vi "TP1.4.vi"() -> ()   [LabVIEW 2013]
panel:
  out "Waveform Graph 2":dbl[](graph)
  in  "Frecuencia":dbl=5.0
  in  "Amplitud":dbl=10.0
  in  "Cantidad de Muestras":i32=1000
  in  "Boolean":bool
  in  "Función":T1(ring)
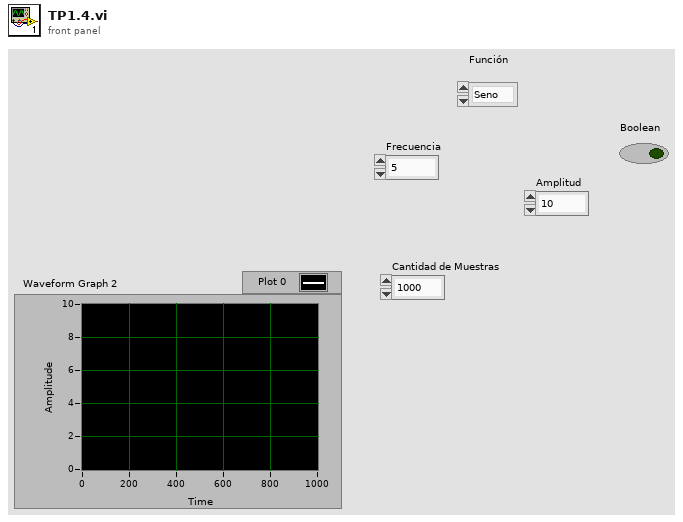
[diagram p1: front panel]
types:
  T1 = enum16{"Seno", "Rampa", "Triangular", "Cuadrada"}
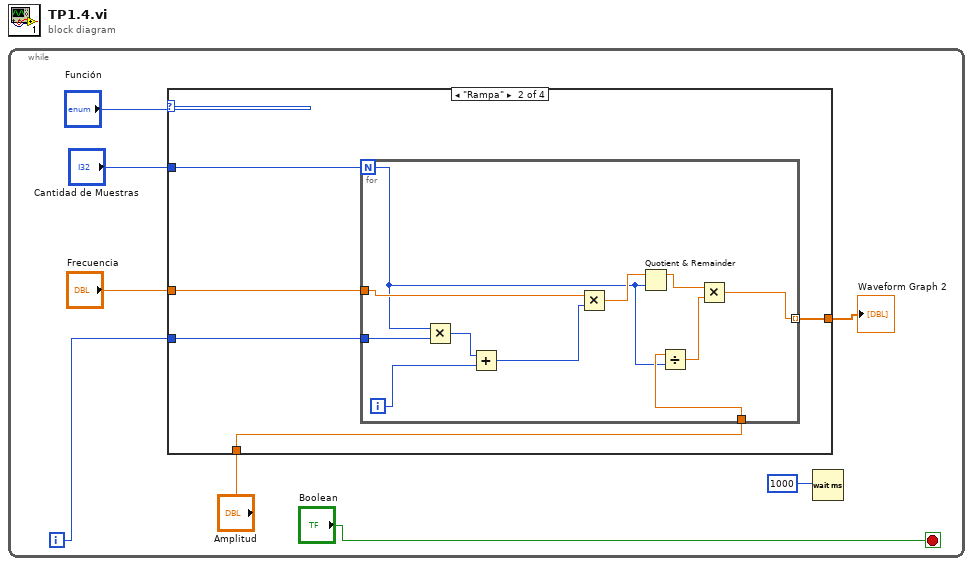
[diagram p0: block diagram]
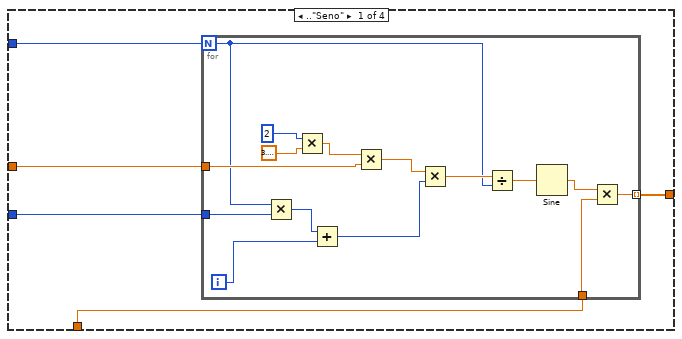
[diagram p2: hidden frame]
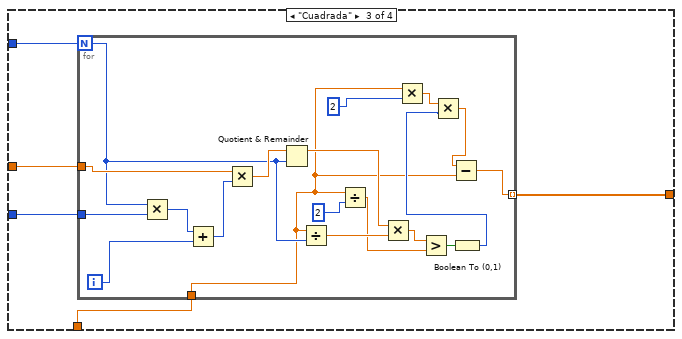
[diagram p3: hidden frame]
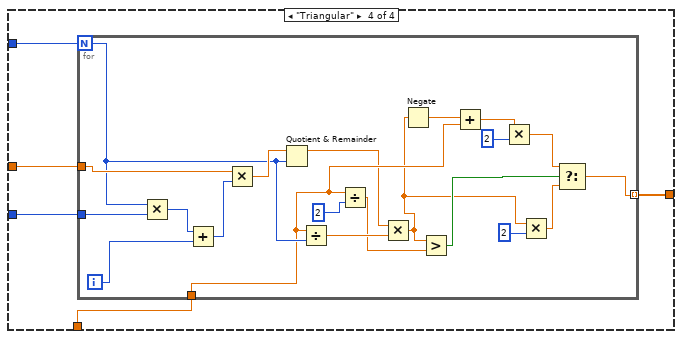
[diagram p4: hidden frame]
diagram:
  n1 = while {
    i -> [w8]
    stop <- "Boolean" stop-if-true
    n2 = case shown="\"Rampa\"" "Función" {
      tunnel: w8 -> [w10 w33 w49 w73]
      tunnel: [w12 w32 w48 w72] -> w6
      tunnel: "Amplitud" -> [w13 w31 w47 w71]
      tunnel: "Cantidad de Muestras" -> [w9 w30 w46 w70]
      tunnel: "Frecuencia" -> [w11 w29 w45 w69]
      frame .."Seno" {
        n3 = for {
          N: w9 -> [w17]
          tunnel: w11 -> [w22]
          tunnel: w13 -> [w21]
          tunnel: [w19] -> w12 mode=indexing
          tunnel: w10 -> [w16]
          i -> [w18]
          n4 = Multiply(x=w17, y=w16) -> (x*y=w15:i32)
          n5 = Multiply(x=2, y=3.141592653589793) -> (x*y=w26:dbl)
          n6 = Add(x=w15, y=w18) -> (x+y=w14:i32)
          n7 = Multiply(x=w26, y=w22) -> (x*y=w25:dbl)
          n8 = Multiply(x=w25, y=w14) -> (x*y=w24:dbl)
          n9 = Divide(x=w24, y=w17) -> (x/y=w23:dbl)
          n10 = Sine(x=w23) -> (sin(x)=w20:dbl)
          n11 = Multiply(x=w20, y=w21) -> (x*y=w19:dbl)
        }
      }
      frame "Rampa" {
        n12 = for {
          N: w30 -> [w37]
          tunnel: w29 -> [w38]
          tunnel: w31 -> [w39]
          tunnel: [w34] -> w32 mode=indexing
          tunnel: w33 -> [w43]
          i -> [w44]
          n13 = Multiply(x=w37, y=w43) -> (x*y=w42:i32)
          n14 = Add(x=w42, y=w44) -> (x+y=w41:i32)
          n15 = Multiply(x=w38, y=w41) -> (x*y=w40:dbl)
          n16 = Quotient & Remainder(x=w40, y=w37) -> (x-y*floor(x/y)=w36:dbl)  [unwired: 1 out]
          n17 = Divide(x=w39, y=w37) -> (x/y=w35:dbl)
          n18 = Multiply(x=w36, y=w35) -> (x*y=w34:dbl)
        }
      }
      frame "Cuadrada" {
        n19 = for {
          N: w46 -> [w62]
          tunnel: w45 -> [w63]
          tunnel: w47 -> [w52]
          tunnel: [w50] -> w48 mode=indexing
          tunnel: w49 -> [w67]
          i -> [w68]
          n20 = Multiply(x=w62, y=w67) -> (x*y=w66:i32)
          n21 = Add(x=w66, y=w68) -> (x+y=w65:i32)
          n22 = Multiply(x=w63, y=w65) -> (x*y=w64:dbl)
          n23 = Quotient & Remainder(x=w64, y=w62) -> (x-y*floor(x/y)=w59:dbl)  [unwired: 1 out]
          n24 = Divide(x=w52, y=w62) -> (x/y=w58:dbl)
          n25 = Divide(x=w52, y=2) -> (x/y=w57:dbl)
          n26 = Multiply(x=w59, y=w58) -> (x*y=w56:dbl)
          n27 = Multiply(x=w52, y=2) -> (x*y=w53:dbl)
          n28 = Greater?(x=w56, y=w57) -> (0:w60:bool)
          n29 = Boolean To (0,1)(Boolean=w60) -> (0, 1=w54:i16)
          n30 = Multiply(x=w53, y=w54) -> (x*y=w51:dbl)
          n31 = Subtract(x=w51, y=w52) -> (x-y=w50:dbl)
        }
      }
      frame "Triangular" {
        n32 = for {
          N: w70 -> [w88]
          tunnel: w69 -> [w89]
          tunnel: w71 -> [w83]
          tunnel: [w82] -> w72 mode=indexing
          tunnel: w73 -> [w93]
          i -> [w94]
          n33 = Multiply(x=w88, y=w93) -> (x*y=w92:i32)
          n34 = Add(x=w92, y=w94) -> (x+y=w91:i32)
          n35 = Multiply(x=w89, y=w91) -> (x*y=w90:dbl)
          n36 = Quotient & Remainder(x=w90, y=w88) -> (x-y*floor(x/y)=w80:dbl)  [unwired: 1 out]
          n37 = Divide(x=w83, y=w88) -> (x/y=w86:dbl)
          n38 = Divide(x=w83, y=2) -> (x/y=w85:dbl)
          n39 = Multiply(x=w80, y=w86) -> (x*y=w75:dbl)
          n40 = Negate(x=w75) -> (-x=w81:dbl)
          n41 = Greater?(x=w75, y=w85) -> (0:w84:bool)
          n42 = Add(x=w81, y=w83) -> (x+y=w79:dbl)
          n43 = Multiply(x=w79, y=2) -> (x*y=w77:dbl)
          n44 = Multiply(x=w75, y=2) -> (x*y=w74:dbl)
          n45 = Select(t=w77, s=w84, f=w74) -> (s? t:f=w82:dbl)
        }
      }
    }
    "Waveform Graph 2" <- w6
    n46 = Wait (ms)(milliseconds to wait=1000) -> ()  [unwired: 1 out]
  }
